vi "Test Process Generate Broadcast Event.vi"(8 "error in (no error)":errorcluster, 11 "Process Test In":refnum<class "Process Dev Test.lvclass">) -> (0 "error out":errorcluster, 3 "Process Test Out":refnum<class "Process Dev Test.lvclass">)   [LabVIEW 2020, in "Process Dev Test.lvclass"]
uses:
  Process Dev Test.lvclass
  source/Framework Test Suite/Mock Process/Mock Process.lvclass
  C:/Git/astemes-triarc-framework/source/Framework/Process/Process.lvclass
  source/Framework/Process/Process.lvclass/Process.ctl
  <vilib>/Astemes/LUnit/Test Case.lvclass/Test Case.ctl
  a972513e-0177-4a2b-a6de-788c1d29ea15.vi
  source/Framework/Process/Public/Lifecycle/Get Lifecycle State.vi
  <vilib>/Astemes/Triarc Framework/Broadcast Event Helpers/Execution timer.vi
  source/Framework/Process/Private/SubVIs/Wait for finish.vi
  source/Framework/Process/Private/SubVIs/Set Lifecycle State.vi
  source/Framework/Process/Protected/Messaging/Send Message.vi
  <vilib>/Astemes/LUnit/Set Assertion Type.vi
  <vilib>/Astemes/LUnit/Palette/Pass.vi
  <vilib>/Astemes/LUnit/Palette/Fail.vi
  <vilib>/Astemes/LUnit/Compare Variants.vi
  <vilib>/Astemes/LUnit/Describe Comparison.vi
  <vilib>/Utility/error.llb/Clear Errors.vi
  source/Framework/Process/Private/SubVIs/Handle Debug Data.vi
  <vilib>/Astemes/LUnit/Add test result.vi
  <vilib>/Astemes/LUnit/Variant to string.vi
  <vilib>/Utility/High Resolution Relative Seconds.vi
  <vilib>/Astemes/LUnit/LUnit Record Assertion Result.vi
  <vilib>/Astemes/LUnit/LUnit Aggregate Assertion Results.vi
  <vilib>/Astemes/LUnit/Method Result/LUnit Merge Status.vi
  <vilib>/Astemes/LUnit/LUnit Concatenate result strings.vi
  <vilib>/Utility/error.llb/Error Cluster From Error Code.vi
  <vilib>/Astemes/Triarc Framework/Broadcast Event Helpers/Dequeue Broadcast Message.vi
  <vilib>/Utility/Data Type/Get Type Information.vi
  <vilib>/Utility/LVClass/Get LV Class Name.vi
  source/Framework/Process/Process.lvclass
  Process Dev Test.lvclass/Process Dev Test.ctl
  <vilib>/Astemes/Triarc Framework/Broadcast Event Helpers/Broadcast Event Helpers.lvlib
  C:/Git/astemes-triarc-framework/source/Framework/Base/Base.lvclass
  C:/Git/astemes-triarc-framework/source/Framework/Configuration File/Configuration File.lvclass
  C:/Git/astemes-triarc-framework/source/Framework/Configuration/Configuration.lvclass
  C:/Git/astemes-triarc-framework/source/Framework/Error Handler Interface/Error Handler Interface.lvclass
  C:/Git/astemes-triarc-framework/source/Framework/Logging/Logging.lvclass
  C:/Git/astemes-triarc-framework/source/Framework Test Suite/Mock Process/Mock Process.lvclass
  C:/Git/astemes-triarc-framework/source/Framework/Async Handler/Async Handler.lvclass
  C:/Git/astemes-triarc-framework/source/Framework/Helper Loop/Helper Loop.lvclass
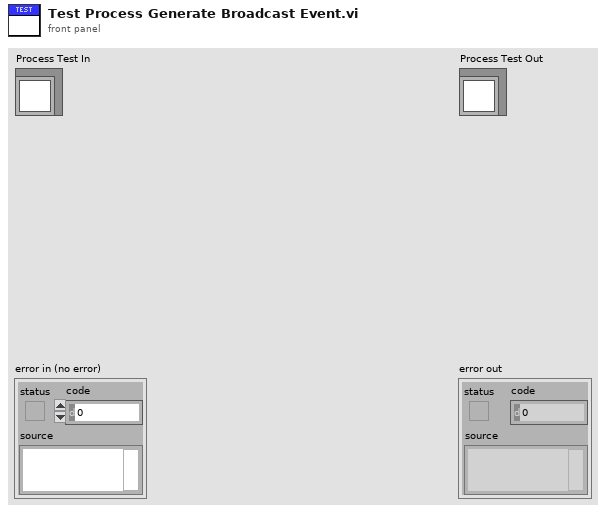
[diagram p1: front panel]
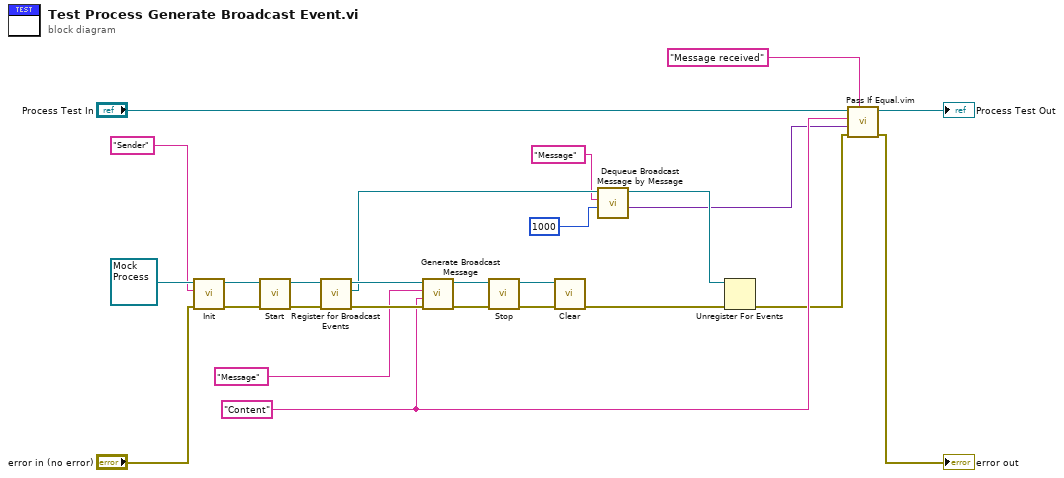
[diagram p0: block diagram]
diagram:
  w11 = "Content" ("Message")
  n1 = call-dynamic "Init.vi"("error in (no error)"="error in (no error)", "Name"="Sender" ("Message"), "Mock Process In"=refnum<class "Mock Process.lvclass"> refnum ("Mock Process.lvclass")) -> ("error out"=w24:errorcluster, "Mock Process Out"=w25:refnum<class "Mock Process.lvclass">)  [unwired: 7 in]
  n2 = call "Start.vi"("error in (no error)"=w24, "Process In"=w25) -> ("error out"=w15:errorcluster, "Process Out"=w17:refnum<class "Mock Process.lvclass">)  [unwired: 7 in, 1 out]
  n3 = call "Register for Broadcast Events.vi"("error in (no error)"=w15, "Process In"=w17) -> ("error out"=w14:errorcluster, "Event Registration Refnum Out"=w13:refnum<event-registration>, "Process Out"=w16:refnum<class "Mock Process.lvclass">)  [unwired: 7 in]
  n4 = call "Generate Broadcast Message.vi"("error in (no error)"=w14, "Message Data"=w11, "Message"="Message", "Mock Process In"=w16) -> ("error out"=w22:errorcluster, "Mock Process Out"=w23:refnum<class "Mock Process.lvclass">)  [unwired: 6 in]
  n5 = call "Stop.vi"("error in (no error)"=w22, "Process In"=w23) -> ("error out"=w21:errorcluster, "Process Out"=w2:refnum<class "Mock Process.lvclass">)  [unwired: 7 in, 1 out]
  n6 = call-dynamic "Clear.vi"("error in (no error)"=w21, "Mock Process In"=w2) -> ("error out"=w20:errorcluster)  [unwired: 9 in]
  n7 = call <vilib>:"Dequeue Broadcast Message by Message.vi"("Timeout (-1)"=1000, "Message"="Message", "Event Registration Refnum"=w13) -> ("Message Data"=w4:variant, "Event Registration Refnum Out"=w12:refnum<event-registration>)  [unwired: 4 in, 3 out]
  n8 = Unregister For Events(event registration refnum=w12, error in=w20) -> (error out=w8:errorcluster)
  n9 = call "Pass If Equal.vim"("Description"="Message received", "error in (no error)"=w8, "Actual"=w4, "Expected"=w11, "LUnit Test Case In"="Process Test In") -> ("error out"=→"error out":errorcluster, "LUnit Test Case Out"=→"Process Test Out":refnum<class "Process Dev Test.lvclass">)  [unwired: 5 in]
